vi "Write Item Type.vi"(8 "error in (no error)":errorcluster, 10 "Item Type":T1, 11 "LabVIEWItem in":refnum<class "LabVIEWItem.lvclass">) -> (0 "error out":errorcluster, 3 "LabVIEWItem out":refnum<class "LabVIEWItem.lvclass">)   [LabVIEW 2019, in "Panther Dashboard.lvlib" / "LabVIEWItem.lvclass"]
uses:
  LabVIEWItem.lvclass
  Item Type--enum.ctl
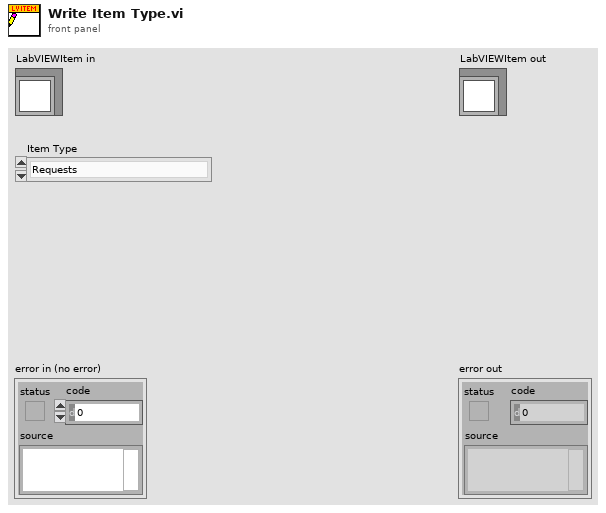
[diagram p1: front panel]
types:
  T1 = typedef "Panther Dashboard.lvlib/LabVIEWItem.lvclass/Item Type--enum.ctl" = enum16{"Requests", "Broadcasts", "Request and Wait for Reply", "Round Trip", "Public API VIs", "» Constant VIs", "» Error VIs", "Module", "Project"}
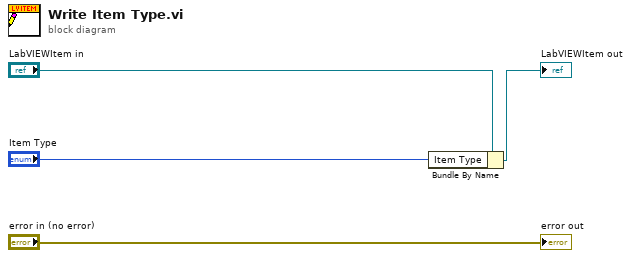
[diagram p0: block diagram]
diagram:
  n1 = Bundle By Name(cluster="LabVIEWItem in", "Item Type"="Item Type") -> (→"LabVIEWItem out":refnum<class "LabVIEWItem.lvclass">)
  "error out" <- "error in (no error)"
